vi "Set relays.vi"(8 "error in (no error)":errorcluster, 10 "System Variables":T1={"Relay 1"="", "Relay 2"="", "Releji"={"Vdd"=0, "GND"=0, "PGD"=0, "PGC"=0, "Reset"=0, "Reference"=""}, "DUT1"=TRUE, "Family name"="", "DUT 2"=FALSE, "DUT test?"=TRUE, "DI0-7"=0, "DI8-15"=0, "DO0-8"=0, "References"={"Relays"=FALSE, "DIO"=FALSE}, "Releji DUT1"={"Vdd"=0, "GND"=0, "PGD"=0, "PGC"=0, "Reset"=0, "Reference"=""}, "Releji DUT2"={"Vdd"=0, "GND"=0, "PGD"=0, "PGC"=0, "Reset"=0, "Reference"=""}}, 11 "ON/OFF":bool) -> (0 "error out":errorcluster)   [LabVIEW 2023]
uses:
  System variables.ctl
  65bd21dc-5c60-413c-9f89-e8b85d79f86b.vi
  Numato/Numato.lvlib
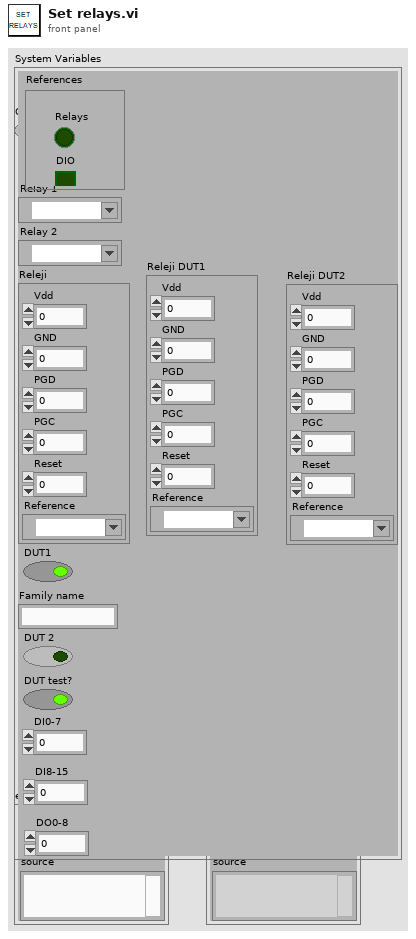
[diagram p1: front panel]
types:
  T1 = typedef "System variables.ctl" = cluster{"Relay 1":refnum<visa-resource-name>, "Relay 2":refnum<visa-resource-name>, "Releji":cluster{"Vdd":i32, "GND":i32, "PGD":i32, "PGC":i32, "Reset":i32, "Reference":refnum<visa-resource-name>}, "DUT1":bool, "Family name":string, "DUT 2":bool, "DUT test?":bool, "DI0-7":i32, "DI8-15":i32, "DO0-8":i32, "References":cluster{"Relays":bool, "DIO":bool}, "Releji DUT1":cluster{"Vdd":i32, "GND":i32, "PGD":i32, "PGC":i32, "Reset":i32, "Reference":refnum<visa-resource-name>}, "Releji DUT2":cluster{"Vdd":i32, "GND":i32, "PGD":i32, "PGC":i32, "Reset":i32, "Reference":refnum<visa-resource-name>}}
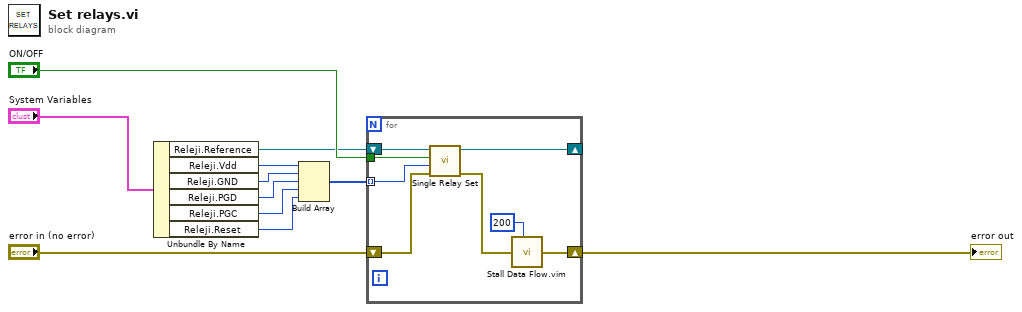
[diagram p0: block diagram]
diagram:
  n1 = Unbundle By Name("System Variables") -> ("Releji.Reference"=w2:refnum<visa-resource-name>, "Releji.Vdd"=w3:i32, "Releji.GND"=w4:i32, "Releji.PGD"=w5:i32, "Releji.PGC"=w6:i32, "Releji.Reset"=w7:i32)
  n2 = Build Array(w3, w4, w5, w6, w7) -> (w8:i32[])
  n3 = for {
    tunnel: w8 -> [w18] mode=indexing
    tunnel: "ON/OFF" -> [w17]
    shift-right: [w13] -> w10
    shift-left: "error in (no error)" -> [w15]
    shift-right: [w14] -> _
    shift-left: w2 -> [w19]
    n4 = call "Single Relay Set.vi"("error in (no error)"=w15, "Relay No"=w18, "ON/OFF"=w17, "VISA resource name"=w19) -> ("error out"=w16:errorcluster, "VISA resource name out"=w14:refnum<visa-resource-name>)  [unwired: 6 in]
    n5 = call "Stall Data Flow.vim"("value in"=w16, "milliseconds to wait"=u32 200) -> ("value out"=w13:errorcluster)  [unwired: 1 out]
  }
  "error out" <- w10
